vi "BlinkM FadeRandomRGB.vi"(0 "Arduino Resource":T1={"VISA resource"="", "Board Type"=enum."Uno", "Connection Type"=enum."USB / Serial", "Bytes Per Packet (15)"=15}, 1 "Address (0)":u8, 2 "Red Variance (0)":u8, 3 "Green Variance (0)":u8, 4 "Blue Variance (0)":u8, 5 "error in":errorcluster) -> (14 "Arduino Resource":T1={"VISA resource"="", "Board Type"=enum."Uno", "Connection Type"=enum."USB / Serial", "Bytes Per Packet (15)"=15}, 19 "error out":errorcluster)   [LabVIEW 2015, in "LabVIEW Interface for Arduino.lvlib"]
doc: "Fade BlinkM to random RGB color in specified range."
uses:
  <vilib>/LabVIEW Interface for Arduino/LabVIEW Interface for Arduino.lvlib
  <vilib>/LabVIEW Interface for Arduino/Type Defs/Arduino Resource.ctl
  <vilib>/LabVIEW Interface for Arduino/Type Defs/Board Type.ctl
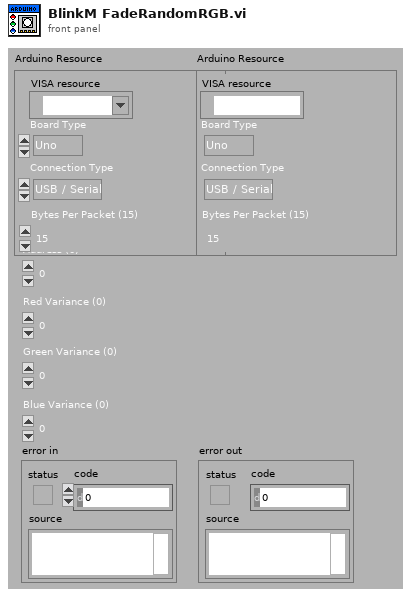
[diagram p1: front panel]
types:
  T1 = typedef "LabVIEW Interface for Arduino.lvlib/Arduino Resource.ctl" = cluster{"VISA resource":refnum<visa-resource-name>, "Board Type":T2, "Connection Type":enum8{"USB / Serial"}, "Bytes Per Packet (15)":u8}
  T2 = typedef "LabVIEW Interface for Arduino.lvlib/Board Type.ctl" = enum16{"Uno", "Dimuelanove w/Atmega 328", "Mega 2560"}
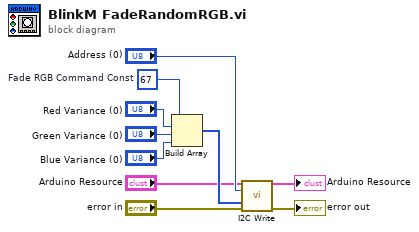
[diagram p0: block diagram]
diagram:
  w7 = u8 67  # Fade RGB Command Const
  n1 = Build Array(w7, "Red Variance (0)", "Green Variance (0)", "Blue Variance (0)") -> (w6:u8[])
  n2 = call <vilib>:"I2C Write.vi"("Arduino Resource"="Arduino Resource", "Address (0)"="Address (0)", "I2C Data Bytes"=w6, "error in"="error in") -> ("Arduino Resource"=→"Arduino Resource":T1, "error out"=→"error out":errorcluster)  [unwired: 10 in]
